vi "Configure Clock 5761.vi"(8 "error in":errorcluster, 10 "Clock Source":T2, 11 "FPGA Interface":T1) -> (0 "error out":errorcluster, 2 "Configuration Error":bool, 3 "FPGA VI Reference Out":T1)   [LabVIEW 2018]
doc: "This VI configures the clock source for the NI 5761. For execution steps, refer to the comments on the block diagram."
uses:
  ClockSource_5761.ctl
  5761 config FPGA ref.ctl
  <vilib>/Utility/error.llb/Error Cluster From Error Code.vi
  <vilib>/rvi/errors/niLvFpgaAdjustHostInterfaceError.vi
  <vilib>/rvi/interface/nirviReadWriteControl/nirviReadWriteControl.xnode
  <vilib>/rvi/interface/Simulation/niFpgaSimulationCallBeginRW.vi
  NiFpgaLv.dll
panel:
  # "This VI configures the clock source for the NI 5761. For execution steps, refer to the comments on the block diagram."
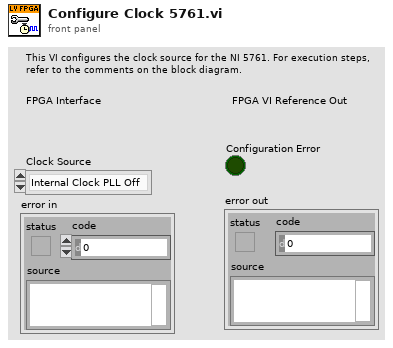
[diagram p1: front panel]
types:
  T1 = typedef "5761 config FPGA ref.ctl" = refnum<k20>
  T2 = typedef "ClockSource_5761.ctl" = enum8{"Internal Clock PLL Off", "Internal Clock PLL On (CLK_IN)", "External Clock (CLK_IN)", "Internal Clock PLL On (IoModSyncClk)", "External Clock (IoModSyncClk)"}
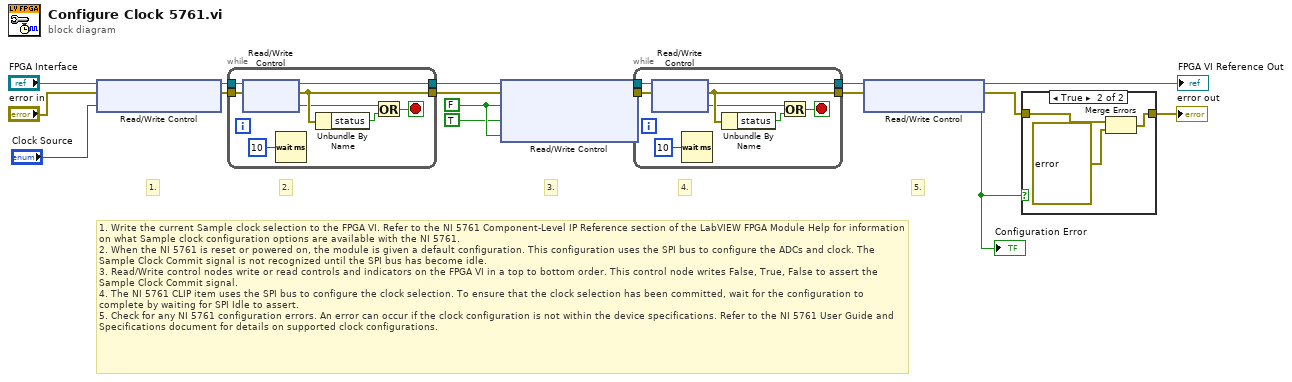
[diagram p0: block diagram]
diagram:
  w9 = FALSE ("Sample Clock Commit")
  # "1. Write the current Sample clock selection to the FPGA VI. Refer to the NI 5761 Component-Level IP Reference section of the LabVIEW FPGA Module Help for information on what Sample clock configuration options are available with the NI 5761.\n2. When the NI 5761 is reset or powered on, the module is given a default configuration. This configuration uses the SPI bus to configure the ADCs and clock. The Sample Clock Commit signal is not recognized until the SPI bus has become idle.\n3. Read/Write control nodes write or read controls and indicators on the FPGA VI in a top to bottom order. This control node writes False, True, False to assert the Sample Clock Commit signal.\n4. The NI 5761 CLIP item uses the SPI bus to configure the clock selection. To ensure that the clock selection has been committed, wait for the configuration to complete by waiting for SPI Idle to assert.\n5. Check for any NI 5761 configuration errors. An error can occur if the clock configuration is not within the device specifications. Refer to the NI 5761 User Guide and Specifications document for details on supported clock configurations."
  # "5."
  # "4."
  # "3."
  # "2."
  # "1."
  n1 = xnode "Read/Write Control"("FPGA VI Reference In"="FPGA Interface", "error in"="error in", "Sample Clock Select"="Clock Source") -> ("FPGA VI Reference Out"=w15:T1, "error out"=w14:errorcluster)
  n2 = while {
    tunnel: w15 -> [w21]
    tunnel: w14 -> [w22]
    tunnel: [w19] -> w12
    tunnel: [w20] -> w13
    stop <- w23 stop-if-true
    n3 = xnode "Read/Write Control"("FPGA VI Reference In"=w21, "error in"=w22) -> ("FPGA VI Reference Out"=w20:T1, "error out"=w19:errorcluster, "SPI Idle"=w18:bool)
    n4 = Wait (ms)(milliseconds to wait=u32 10) -> ()  [unwired: 1 out]
    n5 = Unbundle By Name(w19) -> ("status"=w24:bool)
    n6 = Or(x=w18, y=w24) -> (x .or. y?=w23:bool)
  }
  n7 = xnode "Read/Write Control"("FPGA VI Reference In"=w13, "error in"=w12, "Sample Clock Commit"=w9, "Sample Clock Commit"=TRUE, "Sample Clock Commit"=w9) -> ("FPGA VI Reference Out"=w11:T1, "error out"=w10:errorcluster)
  n8 = while {
    tunnel: w11 -> [w30]
    tunnel: w10 -> [w29]
    tunnel: [w27] -> w6
    tunnel: [w28] -> w7
    stop <- w31 stop-if-true
    n9 = xnode "Read/Write Control"("FPGA VI Reference In"=w30, "error in"=w29) -> ("FPGA VI Reference Out"=w28:T1, "error out"=w27:errorcluster, "SPI Idle"=w26:bool)
    n10 = Wait (ms)(milliseconds to wait=u32 10) -> ()  [unwired: 1 out]
    n11 = Unbundle By Name(w27) -> ("status"=w32:bool)
    n12 = Or(x=w26, y=w32) -> (x .or. y?=w31:bool)
  }
  n13 = xnode "Read/Write Control"("FPGA VI Reference In"=w7, "error in"=w6) -> ("FPGA VI Reference Out"=→"FPGA VI Reference Out":T1, "error out"=w5:errorcluster, "Configuration Error"=w4:bool)
  "Configuration Error" <- w4
  n14 = case shown="True" w4 {
    tunnel: [w34 w37] -> w3
    tunnel: w5 -> [w34 w35]
    frame False {
    }
    frame True {
      n15 = Merge Errors(w35, errorcluster {"status"=TRUE, "code"=-8998, "source"="IO Module clock not configured correctly. Please ensure that the desired clock meets the required specifications."} ("error in")) -> (w37:errorcluster)
    }
  }
  "error out" <- w3
